vi "Read.vi"(8 "error in (no error)":errorcluster, 9 "timeout ms (25000)":i32, 10 "# bytes to read":i32, 11 "dotNET TCP Socket in":refnum<class "dotNET TCP Socket.lvclass">) -> (0 "error out":errorcluster, 2 "Read Bytes":u8[](array[numeric]), 3 "dotNET TCP Socket out":refnum<class "dotNET TCP Socket.lvclass">)   [LabVIEW 2013, in "dotNET SSL Socket.lvlib" / "dotNET TCP Socket.lvclass"]
doc: "Reads data from a socket connection."
uses:
  dotNET TCP Socket.lvclass
  dotNET TCP Socket.lvclass/dotNET TCP Socket.ctl
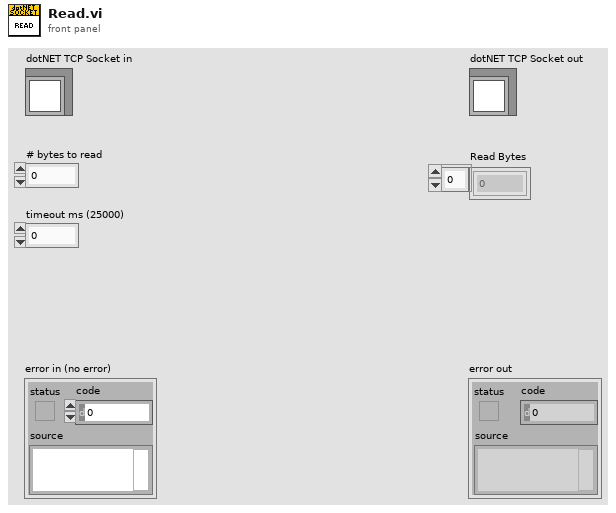
[diagram p1: front panel]
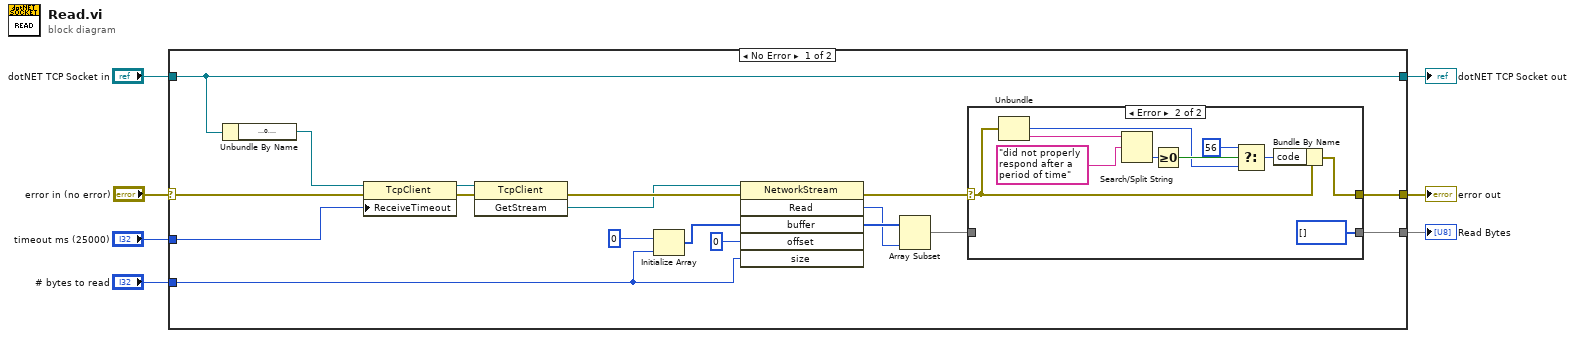
[diagram p0: block diagram]
diagram:
  n1 = case shown="No Error" "error in (no error)" {
    selector: "error in (no error)" -> [w13 w38]
    tunnel: [w18 w38] -> w7
    tunnel: [w17 _] -> w6
    tunnel: "# bytes to read" -> [w16 _]
    tunnel: "timeout ms (25000)" -> [w15 _]
    tunnel: "dotNET TCP Socket in" -> [w12 w39]
    tunnel: [w12 w39] -> w1
    frame No Error {
      n2 = Unbundle By Name(w12) -> ("TcpClient"=w14:refnum<k24>)
      n3 = property class="TcpClient"(reference=w14, error in=w13, "ReceiveTimeout"=w15) -> (reference out=w10:refnum<k24>, error out=w11:errorcluster)
      n4 = invoke class="TcpClient" method="GetStream"(reference=w10, error in=w11) -> (error out=w9:errorcluster, "GetStream"=w8:refnum<k24>)  [unwired: 1 in, 1 out]
      n5 = Initialize Array(u8 0, w16) -> (w24:u8[])
      n6 = invoke class="NetworkStream" method="Read"(reference=w8, error in=w9, "buffer"=w24, "offset"=0, "size"=w16) -> (error out=w20:errorcluster, "Read"=w21:i32, "buffer"=w22:u8[])  [unwired: 1 in, 3 out]
      n7 = Array Subset(array=w22, length=w21) -> (w19:u8[])  [unwired: 1 in]
      n8 = case shown="Error" w20 {
        selector: w20 -> [w27 w33]
        tunnel: [w27 w31] -> w18
        tunnel: [w26 u8[] []] -> w17
        tunnel: w19 -> [w26 _]
        frame No Error {
        }
        frame Error {
          n9 = Unbundle(w33) -> ("code"=w30:i32, "source"=w37:string)  [unwired: 1 out]
          n10 = Search/Split String(string=w37, search string/char (-)="did not properly respond after a period of time") -> (offset of match=w35:i32)  [unwired: 1 in, 2 out]
          n11 = Greater Or Equal To 0?(x=w35) -> (x >= 0?=w34:bool)
          n12 = Select(t=56, s=w34, f=w30) -> (s? t:f=w32:i32)
          n13 = Bundle By Name(cluster=w33, "code"=w32) -> (w31:errorcluster)
        }
      }
    }
    frame Error {
    }
  }
  "error out" <- w7
  "dotNET TCP Socket out" <- w1
  "Read Bytes" <- w6
